vi "main.vi"() -> ()   [LabVIEW 2017]
panel:
  in  "传感器调试":bool
  in  "控制板测试":bool
  in  "传感器评估":bool
  in  "退出":bool
  # "多通道 传感器自动测试系统"
  # "注意：\n传感器评估与参数计算之前，确保已经调试完全，并组装完毕。\n全参数计算之前。请先进行行程测试。\n行程测试为单独测试模块，请独立设置参数。"
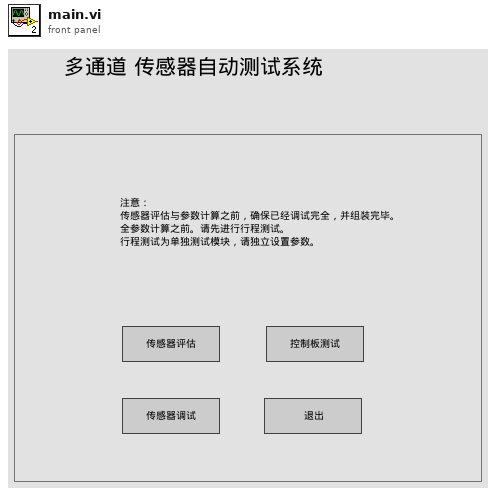
[diagram p1: front panel]
types:
  T1 = enum32{"Invalid", "Standard", "Closed", "Hidden", "Minimized", "Maximized"}
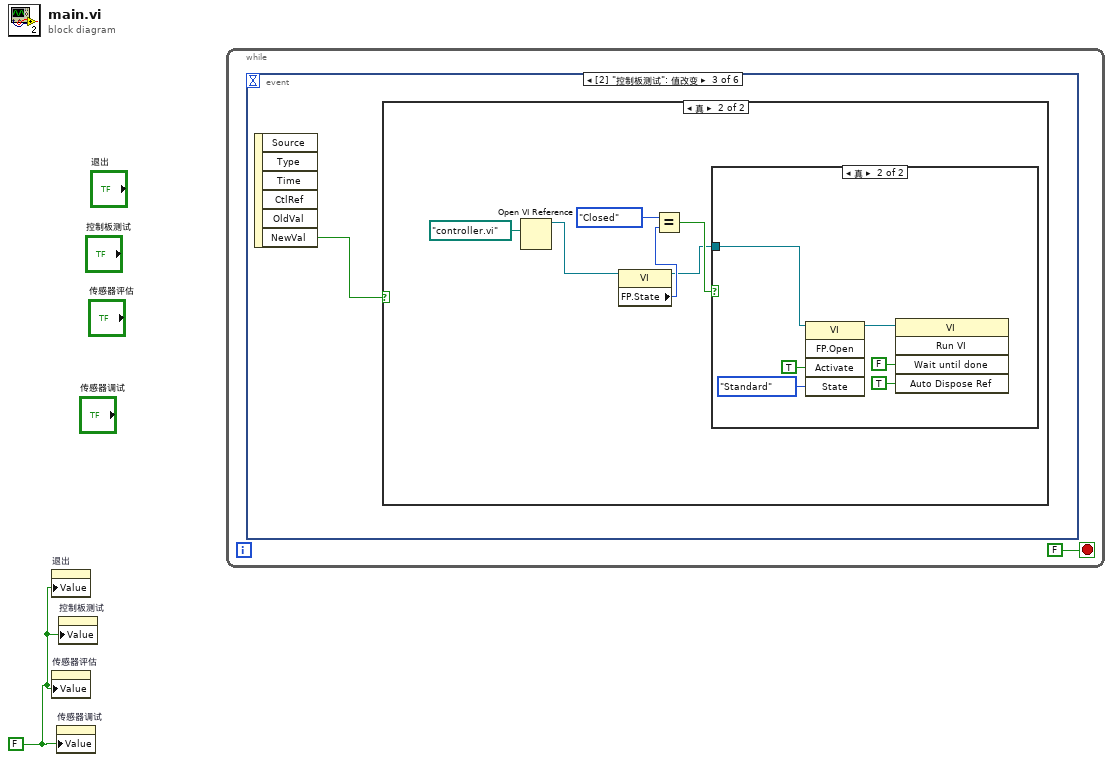
[diagram p0: block diagram]
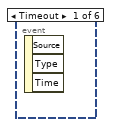
[diagram p2: hidden frame]
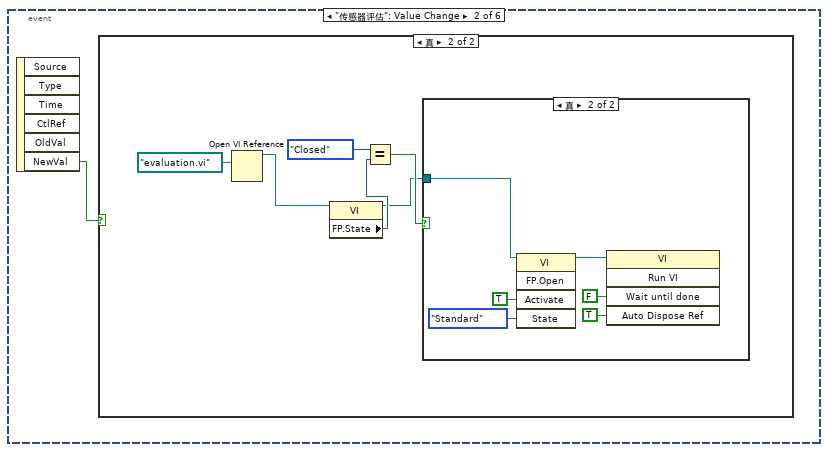
[diagram p3: hidden frame]
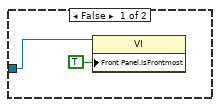
[diagram p5: hidden frame]
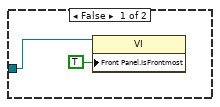
[diagram p7: hidden frame]
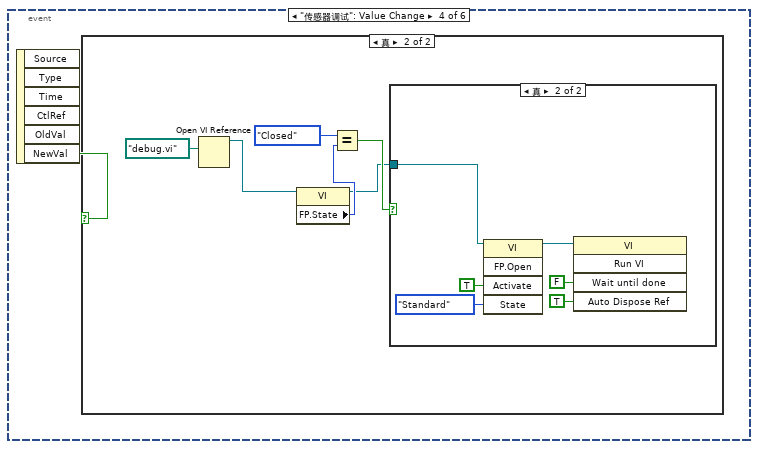
[diagram p8: hidden frame]
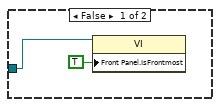
[diagram p10: hidden frame]
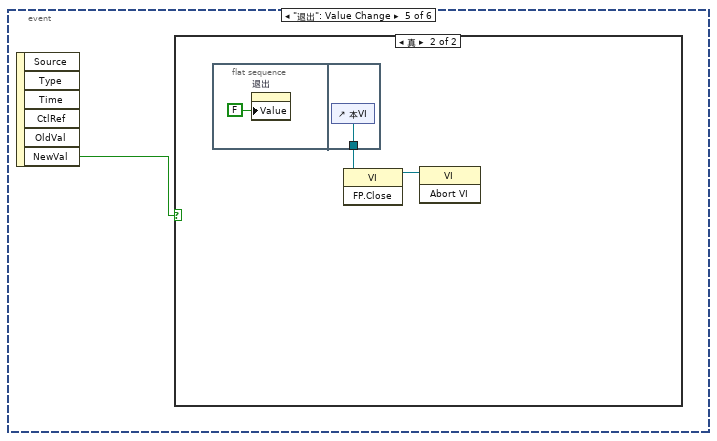
[diagram p11: hidden frame]
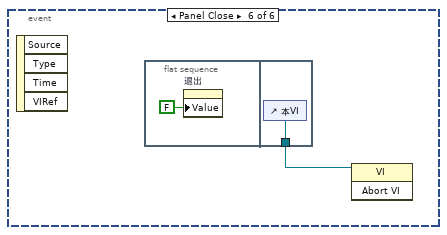
[diagram p13: hidden frame]
diagram:
  w1 = FALSE ("传感器调试")
  n1 = property on="退出" class="Bool (严格)"("Value"=w1) -> ()  [unwired: 2 in, 2 out]
  n2 = property on="传感器评估" class="Bool (严格)"("Value"=w1) -> ()  [unwired: 2 in, 2 out]
  n3 = property on="传感器调试" class="Bool (严格)"("Value"=w1) -> ()  [unwired: 2 in, 2 out]
  n4 = property on="控制板测试" class="Bool (严格)"("Value"=w1) -> ()  [unwired: 2 in, 2 out]
  n5 = while {
    stop <- FALSE stop-if-true
    n6 = event shown="[2] \"控制板测试\": 值改变" {
      selector: _ -> [_ _ _ _ _ _]
      dyn-events: _ -> [_ _ _ _ _ _]
      timeout: _ -> [_ _ _ _ _ _]
      event Timeout {
        n7 = event-data() -> ()  [unwired: 1 in, 3 out]
      }
      event "传感器评估": Value Change {
        n8 = event-data() -> ("NewVal"=w3:bool)  [unwired: 1 in, 5 out]
        n9 = case shown="真" w3 {
          frame False {
          }
          frame True {
            n10 = Open VI Reference(vi path=path "evaluation.vi" ("VI路径")) -> (vi reference=w4:refnum<vi>)  [unwired: 5 in, 1 out]
            n11 = property class="VI"(reference=w4) -> (reference out=w5:refnum<vi>, "FP.State"=w8:T1)  [unwired: 1 in, 1 out]
            n12 = Equal?(x=T1."Closed", y=w8) -> (x = y?=w6:bool)
            n13 = case shown="真" w6 {
              tunnel: w5 -> [w10 w12]
              frame False {
                n14 = property class="VI"(reference=w10, "Front Panel.IsFrontmost"=TRUE ("前面板窗口:在最前")) -> ()  [unwired: 1 in, 2 out]
              }
              frame True {
                n15 = invoke class="VI" method="FP.Open"(reference=w12, "Activate"=TRUE ("激活？"), "State"=T1."Standard" ("状态")) -> (reference out=w15:refnum<vi>)  [unwired: 2 in, 4 out]
                n16 = invoke class="VI" method="Run VI"(reference=w15, "Wait until done"=FALSE ("结束前等待"), "Auto Dispose Ref"=TRUE ("自动销毁引用")) -> ()  [unwired: 2 in, 5 out]
              }
            }
          }
        }
      }
      event "控制板测试": Value Change {
        n17 = event-data() -> ("NewVal"=w18:bool)  [unwired: 1 in, 5 out]
        n18 = case shown="真" w18 {
          frame False {
          }
          frame True {
            n19 = Open VI Reference(vi path=path "controller.vi" ("VI路径")) -> (vi reference=w19:refnum<vi>)  [unwired: 5 in, 1 out]
            n20 = property class="VI"(reference=w19) -> (reference out=w20:refnum<vi>, "FP.State"=w23:T1)  [unwired: 1 in, 1 out]
            n21 = Equal?(x=T1."Closed", y=w23) -> (x = y?=w21:bool)
            n22 = case shown="真" w21 {
              tunnel: w20 -> [w25 w27]
              frame False {
                n23 = property class="VI"(reference=w25, "Front Panel.IsFrontmost"=TRUE ("前面板窗口:在最前")) -> ()  [unwired: 1 in, 2 out]
              }
              frame True {
                n24 = invoke class="VI" method="FP.Open"(reference=w27, "Activate"=TRUE ("激活？"), "State"=T1."Standard" ("状态")) -> (reference out=w30:refnum<vi>)  [unwired: 2 in, 4 out]
                n25 = invoke class="VI" method="Run VI"(reference=w30, "Wait until done"=FALSE ("结束前等待"), "Auto Dispose Ref"=TRUE ("自动销毁引用")) -> ()  [unwired: 2 in, 5 out]
              }
            }
          }
        }
      }
      event "传感器调试": Value Change {
        n26 = event-data() -> ("NewVal"=w33:bool)  [unwired: 1 in, 5 out]
        n27 = case shown="真" w33 {
          frame False {
          }
          frame True {
            n28 = Open VI Reference(vi path=path "debug.vi" ("VI路径")) -> (vi reference=w34:refnum<vi>)  [unwired: 5 in, 1 out]
            n29 = property class="VI"(reference=w34) -> (reference out=w35:refnum<vi>, "FP.State"=w38:T1)  [unwired: 1 in, 1 out]
            n30 = Equal?(x=T1."Closed", y=w38) -> (x = y?=w36:bool)
            n31 = case shown="真" w36 {
              tunnel: w35 -> [w40 w42]
              frame False {
                n32 = property class="VI"(reference=w40, "Front Panel.IsFrontmost"=TRUE ("前面板窗口:在最前")) -> ()  [unwired: 1 in, 2 out]
              }
              frame True {
                n33 = invoke class="VI" method="FP.Open"(reference=w42, "Activate"=TRUE ("激活？"), "State"=T1."Standard" ("状态")) -> (reference out=w45:refnum<vi>)  [unwired: 2 in, 4 out]
                n34 = invoke class="VI" method="Run VI"(reference=w45, "Wait until done"=FALSE ("结束前等待"), "Auto Dispose Ref"=TRUE ("自动销毁引用")) -> ()  [unwired: 2 in, 5 out]
              }
            }
          }
        }
      }
      event "退出": Value Change {
        n35 = event-data() -> ("NewVal"=w48:bool)  [unwired: 1 in, 5 out]
        n36 = case shown="真" w48 {
          frame False {
          }
          frame True {
            n37 = flat-sequence {
              tunnel: [w52] -> w50
              frame #0 {
                n38 = property on="退出" class="Bool (严格)"("Value"=FALSE ("退出")) -> ()  [unwired: 2 in, 2 out]
              }
              frame #1 {
                n39 = control-ref of="本VI"() -> (w52:refnum<vi>)
              }
            }
            n40 = invoke class="VI" method="FP.Close"(reference=w50) -> (reference out=w49:refnum<vi>)  [unwired: 2 in, 2 out]
            n41 = invoke class="VI" method="Abort VI"(reference=w49) -> ()  [unwired: 2 in, 3 out]
          }
        }
      }
      event Panel Close {
        n42 = event-data() -> ()  [unwired: 1 in, 4 out]
        n43 = flat-sequence {
          tunnel: [w55] -> w53
          frame #0 {
            n44 = property on="退出" class="Bool (严格)"("Value"=FALSE ("退出")) -> ()  [unwired: 2 in, 2 out]
          }
          frame #1 {
            n45 = control-ref of="本VI"() -> (w55:refnum<vi>)
          }
        }
        n46 = invoke class="VI" method="Abort VI"(reference=w53) -> ()  [unwired: 2 in, 3 out]
      }
    }
  }
